vi "load_xml.vi"(8 "error in":errorcluster, 10 "child node in":refnum<k20>) -> (0 "error out":errorcluster, 2 "child node out":refnum<k20>, 3 "Variable Settings":T1={"Measurements per Iteration"=1, "Local Data Path"=path "C:/Users/Saffmanlab/Documents/Cesium/data", "Experiment description suffix for filename (no spaces please)"="", "Network Data Path"=path "Z:/", "Copy data to network"=TRUE, "Measurement Timeout (ms)"=0, "Independent Variables"=[], "Dependent Variables"=[], "Run Test Mode"=FALSE} {"Independent Variables"."# steps" min=1 step=1; "Measurements per Iteration" min=1 step=1})   [LabVIEW 2013, in "ExperimentVariables.lvclass"]
doc: "This .vi load in data from a saved .xml file for the Experiment Variables section of the settings.\n\nThe expected format is:\n\n<IndependentVariables columns=\"Description,Name (a,a0...a9),min,max,# steps\">\n<var>%s\\t%s\\t%f\\t%f\\t%u</var>\n</IndependentVariables>\n<DependentVariables columns=\"Description,Name (a,a0...a9),Equation,Result\">\n<var>%s\\t%s\\t%s\\t%f</var>\n</DependentVariables>\n<MeasurementsPerIteration>%u</MeasurementsPerIteration>\n<LocalDataPath>%s</LocalDataPath>\n<ExperimentDescriptionSuffix>%s</ExperimentDescriptionSuffix>\n<NetworkDataPath>%s</NetworkDataPath>\n<CopyDataToNetwork>%b</CopyDataToNetwork>\n<MeasurementTimeout units=\"ms\">%u</MeasurementTimeout>\n<RunTestMode>%b</RunTestMode>\n\nMTL 2013 Jan 1"
uses:
  ExperimentVariables.lvclass
  Variable_Settings.ctl
  <vilib>/xml/Close Reference(Node).vi
  <resource>/objmgr/DOMUserDefRef.rc
  <vilib>/xml/NI_XML.lvlib
panel:
  # "Parameters will be evaluated once at the beginning of the experiment from top to bottom, \nso any parameter may depend on all those above it.\nVariables will be evaluated each iteration.\nParameters and Variables may be used in various other experiment settings, as noted.\nSee LabView Help -> Formula Node and Expression Node Functions for a list of available functions."
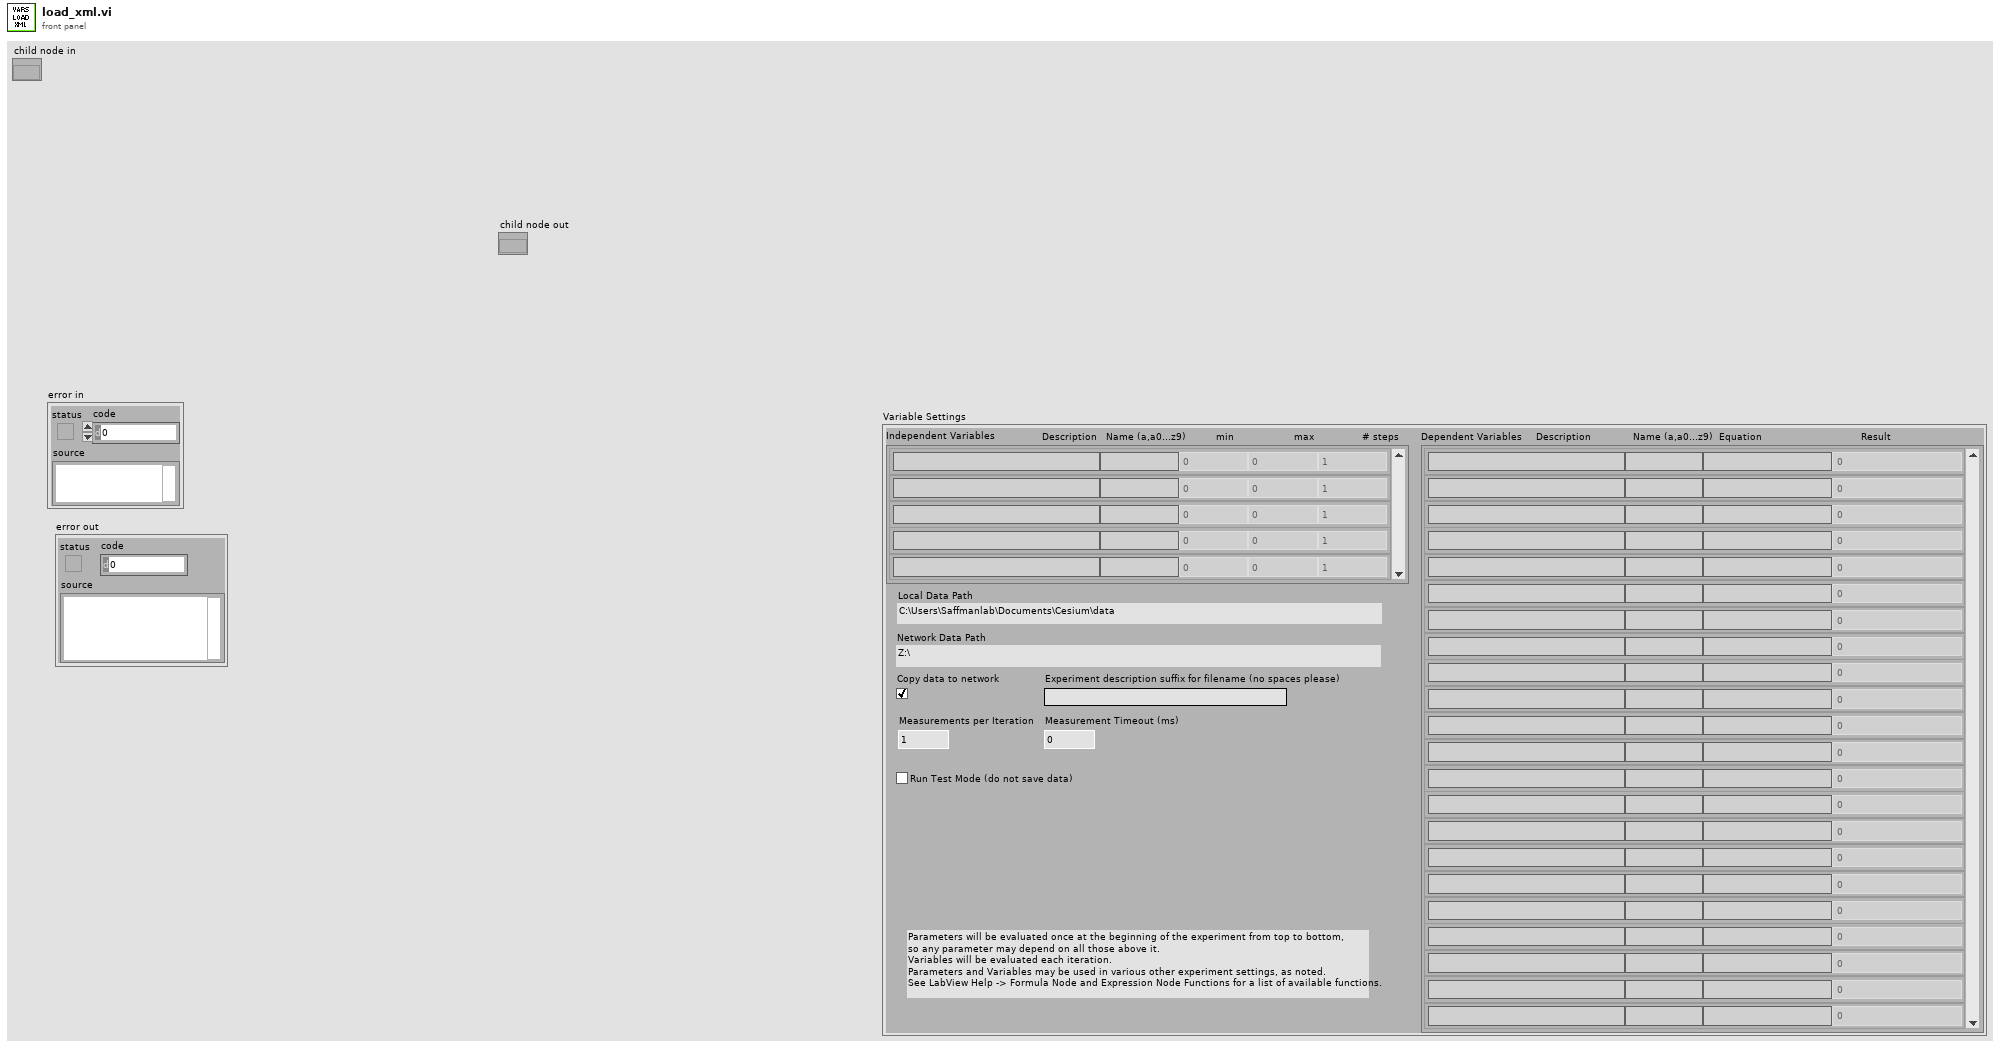
[diagram p1: front panel]
types:
  T1 = typedef "ExperimentVariables.lvclass/Variable_Settings.ctl" = cluster{"Measurements per Iteration":i32, "Local Data Path":path, "Experiment description suffix for filename (no spaces please)":string, "Network Data Path":path, "Copy data to network":bool, "Measurement Timeout (ms)":u32, "Independent Variables":cluster{"Description":string, "Name (a,a0...a9)":string, "min":dbl, "max":dbl, "# steps":u32}[], "Dependent Variables":cluster{"Description":string, "Name (a,a0...a9)":string, "Equation":string, "Result":dbl}[], "Run Test Mode":bool}
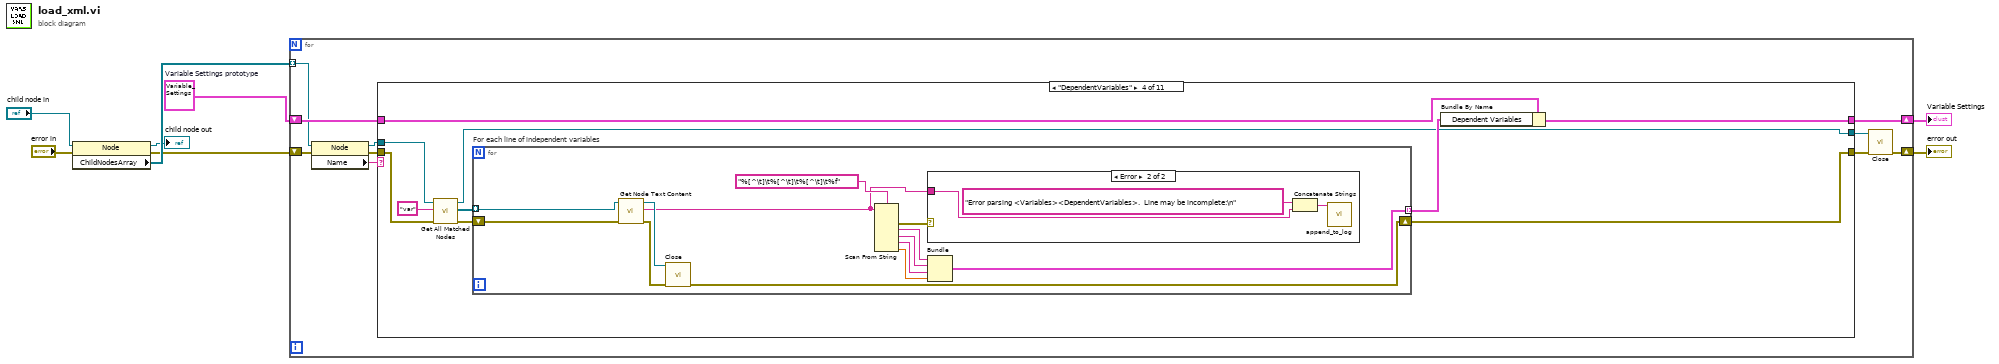
[diagram p0: block diagram]
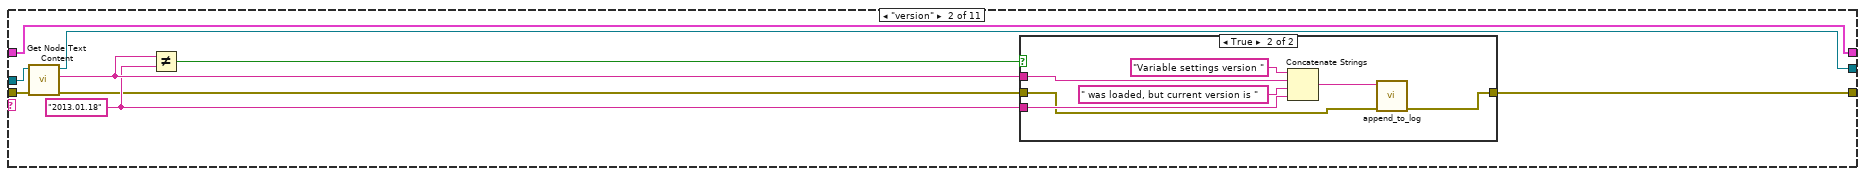
[diagram p3: hidden frame]
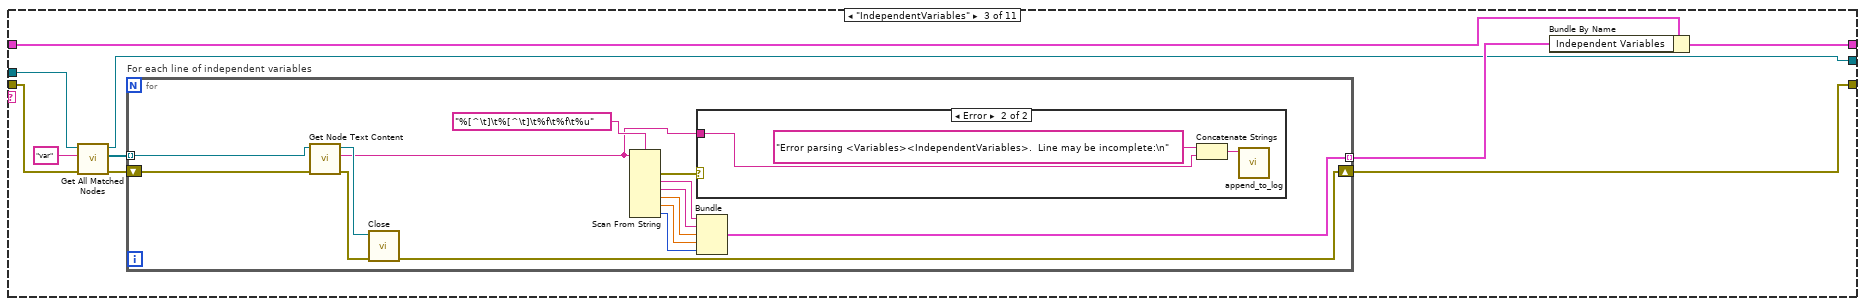
[diagram p5: hidden frame]
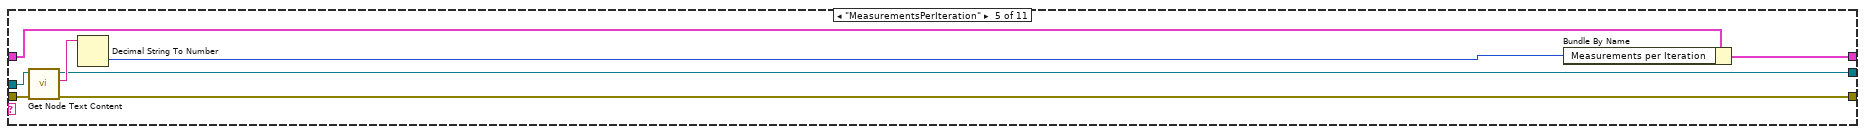
[diagram p8: hidden frame]
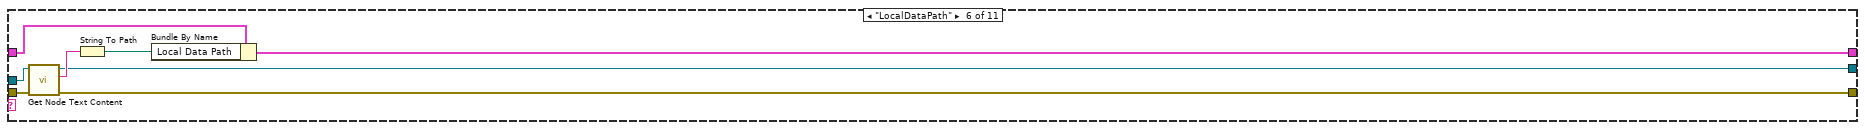
[diagram p9: hidden frame]
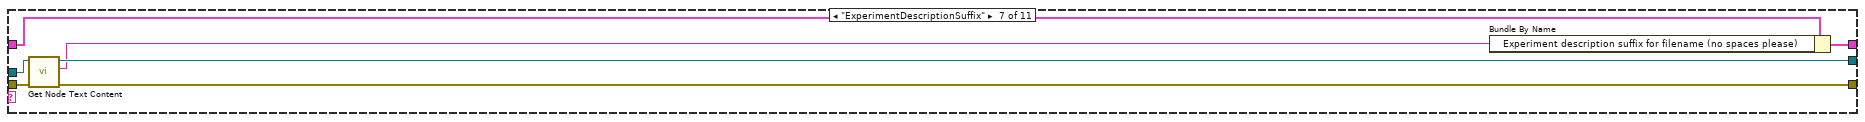
[diagram p10: hidden frame]
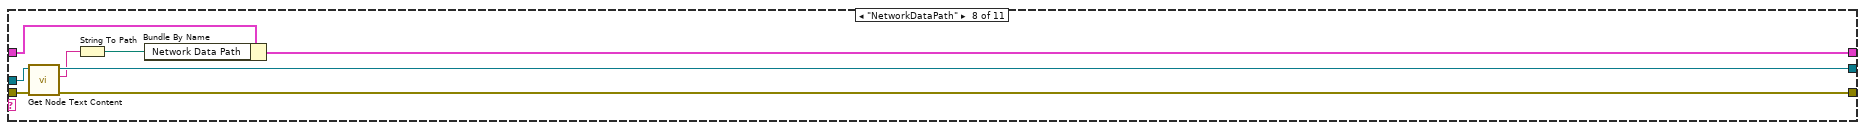
[diagram p11: hidden frame]
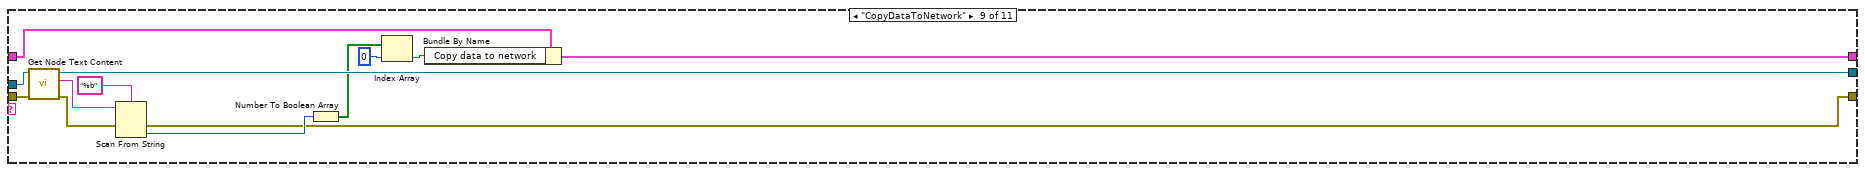
[diagram p12: hidden frame]
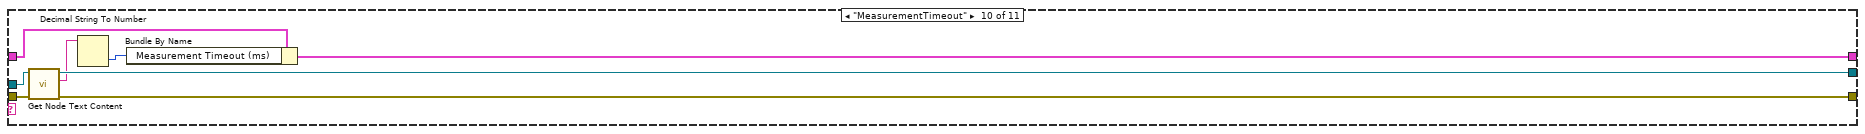
[diagram p13: hidden frame]
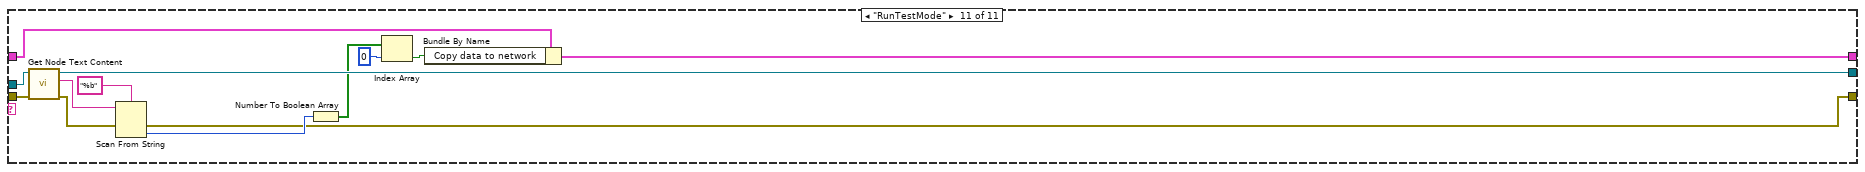
[diagram p14: hidden frame]
diagram:
  w7 = T1 {"Measurements per Iteration"=1, "Local Data Path"=path "C:/Users/Saffmanlab/Documents/Cesium/data", "Experiment description suffix for filename (no spaces please)"="", "Network Data Path"=path "Z:/", "Copy data to network"=TRUE, "Measurement Timeout (ms)"=0, "Independent Variables"=[], "Dependent Variables"=[], "Run Test Mode"=FALSE}  # Variable Settings prototype
  n1 = property class="Node"(reference="child node in", error in="error in") -> (reference out=→"child node out":refnum<k20>, error out=w3:errorcluster, "ChildNodesArray"=w8:refnum<k20>[])
  n2 = for {
    tunnel: w8 -> [w9] mode=indexing
    shift-right: [w15] -> w5
    shift-left: w7 -> [w16]
    shift-right: [w12] -> w2
    shift-left: w3 -> [w10]
    n3 = property class="Node"(reference=w9, error in=w10) -> (reference out=w17:refnum<k20>, error out=w13:errorcluster, "Name"=w18:string)
    n4 = case shown="\"DependentVariables\"" w18 {
      tunnel: w17 -> [w20 w26 w48 w75 w95 w102 w111 w119 w132 w140 w155]
      tunnel: w16 -> [w21 w22 w45 w72 w99 w107 w114 w122 w135 w143 w145]
      tunnel: [w21 w22 w43 w70 w98 w106 w113 w121 w134 w142 w144] -> w15
      tunnel: [w20 w24 w42 w69 w94 w103 w112 w120 w133 w141 w156] -> w14
      tunnel: w13 -> [w19 w25 w41 w68 w93 w101 w110 w118 w131 w139 w154]
      tunnel: [w19 w23 w39 w66 w92 w100 w109 w117 w123 w136 w146] -> w11
      frame "None", Default {
      }
      frame "version" {
        w28 = "2013.01.18" ("y")
        n5 = call <vilib>:"Get Node Text Content.vi"("error in (no error)"=w25, "node in"=w26) -> ("error out"=w27:errorcluster, "node text"=w29:string, "node out"=w24:refnum<k20>)  [unwired: 7 in]
        n6 = Not Equal?(x=w29, y=w28) -> (x != y?=w30:bool)
        n7 = case shown="True" w30 {
          tunnel: w29 -> [_ w37]
          tunnel: w28 -> [_ w35]
          tunnel: w27 -> [w31 w33]
          tunnel: [w31 w32] -> w23
          frame False {
          }
          frame True {
            n8 = Concatenate Strings("Variable settings version " ("string"), w37, " was loaded, but current version is " ("string"), w35) -> (w34:string)
            n9 = call "append_to_log.vi"("error in"=w33, "string"=w34) -> ("error out"=w32:errorcluster)  [unwired: 9 in]
          }
        }
      }
      frame "IndependentVariables" {
        n10 = call <vilib>:"Get All Matched Nodes.vi"("error in (no error)"=w41, "XPath expression"="var", "node in"=w48) -> ("error out"=w40:errorcluster, "node result array"=w46:refnum<k20>[], "node out"=w42:refnum<k20>)  [unwired: 6 in]
        n11 = for "For each line of independent variables" {
          tunnel: w46 -> [w57] mode=indexing
          tunnel: [w58] -> w44 mode=indexing
          shift-right: [w52] -> w39
          shift-left: w40 -> [w53]
          n12 = call <vilib>:"Get Node Text Content.vi"("error in (no error)"=w53, "node in"=w57) -> ("error out"=w51:errorcluster, "node text"=w49:string, "node out"=w54:refnum<k20>)  [unwired: 7 in]
          n13 = call-poly <vilib>:"Close.vi"("error in (no error)"=w51, "node"=w54) -> ("error out"=w52:errorcluster)  [unwired: 7 in]
          n14 = Scan From String(format string="%[^\t]\t%[^\t]\t%f\t%f\t%u", input string=w49) -> (error out=w50:errorcluster, output 1=w56:string, output 2=w55:string, output 3=w61:dbl, output 4=w60:dbl, output 5=w59:u32)  [unwired: 7 in, 2 out]
          n15 = case shown="Error" w50 {
            tunnel: w49 -> [_ w63]
            frame No Error {
            }
            frame Error {
              n16 = Concatenate Strings("Error parsing <Variables><IndependentVariables>.  Line may be incomplete:\n" ("string"), w63) -> (w64:string)
              n17 = call "append_to_log.vi"("string"=w64) -> ()  [unwired: 10 in, 1 out]
            }
          }
          n18 = Bundle(w56, w55, w61, w60, w59) -> (w58:cluster{string, string, dbl, dbl, u32})  [unwired: 1 in]
        }
        n19 = Bundle By Name(cluster=w45, "Independent Variables"=w44) -> (w43:T1)
      }
      frame "DependentVariables" {
        n20 = call <vilib>:"Get All Matched Nodes.vi"("error in (no error)"=w68, "XPath expression"="var", "node in"=w75) -> ("error out"=w67:errorcluster, "node result array"=w73:refnum<k20>[], "node out"=w69:refnum<k20>)  [unwired: 6 in]
        n21 = for "For each line of independent variables" {
          tunnel: w73 -> [w84] mode=indexing
          tunnel: [w85] -> w71 mode=indexing
          shift-right: [w79] -> w66
          shift-left: w67 -> [w80]
          n22 = call <vilib>:"Get Node Text Content.vi"("error in (no error)"=w80, "node in"=w84) -> ("error out"=w78:errorcluster, "node text"=w76:string, "node out"=w81:refnum<k20>)  [unwired: 7 in]
          n23 = call-poly <vilib>:"Close.vi"("error in (no error)"=w78, "node"=w81) -> ("error out"=w79:errorcluster)  [unwired: 7 in]
          n24 = Scan From String(format string="%[^\t]\t%[^\t]\t%[^\t]\t%f", input string=w76) -> (error out=w77:errorcluster, output 1=w83:string, output 2=w82:string, output 3=w87:string, output 4=w86:dbl)  [unwired: 6 in, 2 out]
          n25 = case shown="Error" w77 {
            tunnel: w76 -> [_ w89]
            frame No Error {
            }
            frame Error {
              n26 = Concatenate Strings("Error parsing <Variables><DependentVariables>.  Line may be incomplete:\n" ("string"), w89) -> (w90:string)
              n27 = call "append_to_log.vi"("string"=w90) -> ()  [unwired: 10 in, 1 out]
            }
          }
          n28 = Bundle(w83, w82, w87, w86) -> (w85:cluster{string, string, string, dbl})  [unwired: 1 in]
        }
        n29 = Bundle By Name(cluster=w72, "Dependent Variables"=w71) -> (w70:T1)
      }
      frame "MeasurementsPerIteration" {
        n30 = call <vilib>:"Get Node Text Content.vi"("error in (no error)"=w93, "node in"=w95) -> ("error out"=w92:errorcluster, "node text"=w97:string, "node out"=w94:refnum<k20>)  [unwired: 7 in]
        n31 = Decimal String To Number(string=w97) -> (number=w96:i32)  [unwired: 2 in, 1 out]
        n32 = Bundle By Name(cluster=w99, "Measurements per Iteration"=w96) -> (w98:T1)
      }
      frame "LocalDataPath" {
        n33 = call <vilib>:"Get Node Text Content.vi"("error in (no error)"=w101, "node in"=w102) -> ("error out"=w100:errorcluster, "node text"=w105:string, "node out"=w103:refnum<k20>)  [unwired: 7 in]
        n34 = String To Path(string=w105) -> (path=w104:path)
        n35 = Bundle By Name(cluster=w107, "Local Data Path"=w104) -> (w106:T1)
      }
      frame "ExperimentDescriptionSuffix" {
        n36 = call <vilib>:"Get Node Text Content.vi"("error in (no error)"=w110, "node in"=w111) -> ("error out"=w109:errorcluster, "node text"=w108:string, "node out"=w112:refnum<k20>)  [unwired: 7 in]
        n37 = Bundle By Name(cluster=w114, "Experiment description suffix for filename (no spaces please)"=w108) -> (w113:T1)
      }
      frame "NetworkDataPath" {
        n38 = call <vilib>:"Get Node Text Content.vi"("error in (no error)"=w118, "node in"=w119) -> ("error out"=w117:errorcluster, "node text"=w116:string, "node out"=w120:refnum<k20>)  [unwired: 7 in]
        n39 = String To Path(string=w116) -> (path=w115:path)
        n40 = Bundle By Name(cluster=w122, "Network Data Path"=w115) -> (w121:T1)
      }
      frame "CopyDataToNetwork" {
        n41 = call <vilib>:"Get Node Text Content.vi"("error in (no error)"=w131, "node in"=w132) -> ("error out"=w124:errorcluster, "node text"=w126:string, "node out"=w133:refnum<k20>)  [unwired: 7 in]
        n42 = Scan From String(format string="%b", input string=w126, error in=w124) -> (error out=w123:errorcluster, output 1=w125:i32)  [unwired: 2 in, 2 out]
        n43 = Number To Boolean Array(number=w125) -> (Boolean array=w130:bool[])
        n44 = Index Array(array=w130, index=0) -> (element=w128:bool)
        n45 = Bundle By Name(cluster=w135, "Copy data to network"=w128) -> (w134:T1)
      }
      frame "MeasurementTimeout" {
        n46 = call <vilib>:"Get Node Text Content.vi"("error in (no error)"=w139, "node in"=w140) -> ("error out"=w136:errorcluster, "node text"=w138:string, "node out"=w141:refnum<k20>)  [unwired: 7 in]
        n47 = Decimal String To Number(string=w138) -> (number=w137:i32)  [unwired: 2 in, 1 out]
        n48 = Bundle By Name(cluster=w143, "Measurement Timeout (ms)"=w137) -> (w142:T1)
      }
      frame "RunTestMode" {
        n49 = call <vilib>:"Get Node Text Content.vi"("error in (no error)"=w154, "node in"=w155) -> ("error out"=w147:errorcluster, "node text"=w148:string, "node out"=w156:refnum<k20>)  [unwired: 7 in]
        n50 = Scan From String(format string="%b", input string=w148, error in=w147) -> (error out=w146:errorcluster, output 1=w149:i32)  [unwired: 2 in, 2 out]
        n51 = Number To Boolean Array(number=w149) -> (Boolean array=w153:bool[])
        n52 = Index Array(array=w153, index=0) -> (element=w151:bool)
        n53 = Bundle By Name(cluster=w145, "Copy data to network"=w151) -> (w144:T1)
      }
    }
    n54 = call-poly <vilib>:"Close.vi"("error in (no error)"=w11, "node"=w14) -> ("error out"=w12:errorcluster)  [unwired: 7 in]
  }
  "error out" <- w2
  "Variable Settings" <- w5
